vi "Name Msg IO.vi"(4 "IO":T4, 6 "Name Msg":string, 8 "error in":errorcluster, 9 "Name Library File Path":path, 10 "Active Project":refnum<vi>) -> (0 "error out":errorcluster, 2 "Name Msg IO":T1)   [LabVIEW 2025, in "_Rescript.lvlib" / "Msg.lvlib" / "Msg.lvclass"]
uses:
  Msg.lvclass
  IO.ctl
  Name Msg IO.ctl
  Terminal Attributes.ctl
  Attributes.ctl
  <vilib>/Utility/traverseref.llb/TRef TravTarget.ctl
  _Rescript.lvlib
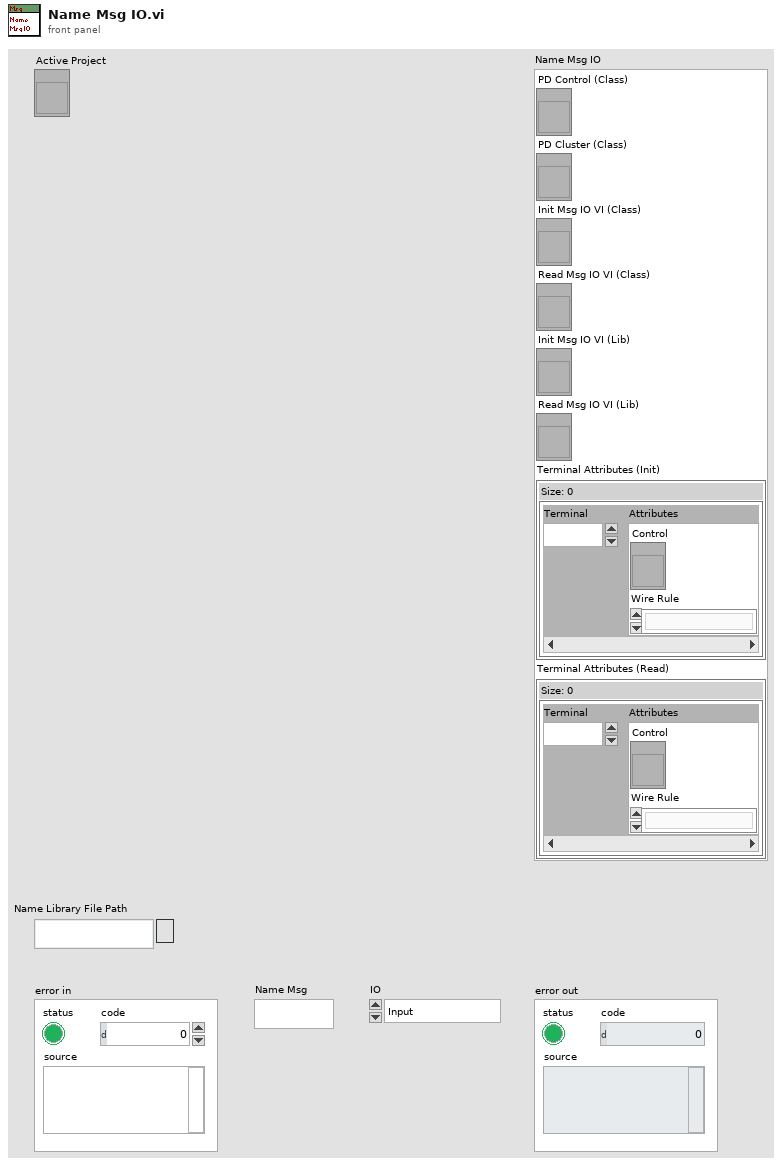
[diagram p1: front panel]
types:
  T1 = typedef "_Rescript.lvlib/Msg.lvlib/Msg.lvclass/Name Msg IO.ctl" = cluster{"PD Control (Class)":refnum<vi>, "PD Cluster (Class)":refnum<vi>, "Init Msg IO VI (Class)":refnum<vi>, "Read Msg IO VI (Class)":refnum<vi>, "Init Msg IO VI (Lib)":refnum<vi>, "Read Msg IO VI (Lib)":refnum<vi>, "Terminal Attributes (Init)":T2, "Terminal Attributes (Read)":T2}
  T2 = typedef "_Rescript.lvlib/Terminal Attributes.ctl" = map{i32, T3}
  T3 = typedef "_Rescript.lvlib/Attributes.ctl" = cluster{"Control":refnum<vi>, "Wire Rule":enum16{"Invalid Wire Rule", "Required", "Recommended", "Optional", "Dynamic Dispatch"}}
  T4 = typedef "_Rescript.lvlib/Msg.lvlib/Msg.lvclass/IO.ctl" = enum16{"Input", "Output"}
  T5 = typedef "TRef TravTarget.ctl" = enum16{"FP", "BD", "Other"}
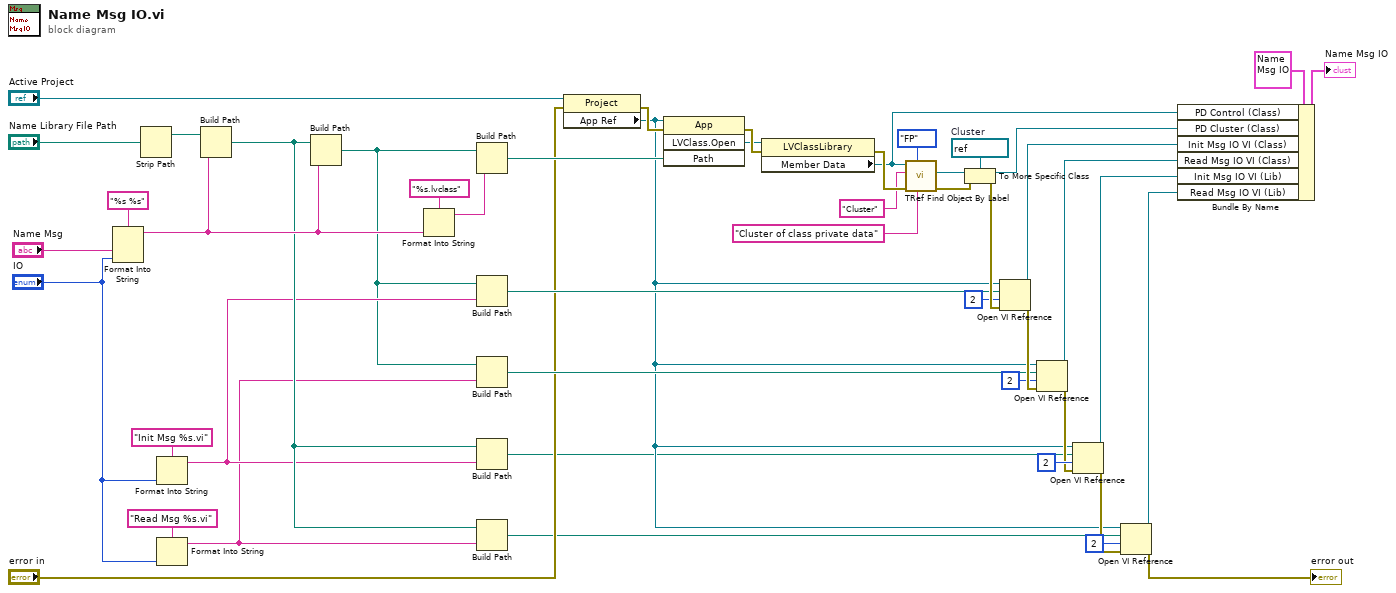
[diagram p0: block diagram]
diagram:
  w43 = refnum<vi> refnum  # Cluster
  n1 = Format Into String(format string="%s %s", "Name Msg", "IO") -> (resulting string=w7:string)  [unwired: 2 in, 1 out]
  n2 = Strip Path(path="Name Library File Path") -> (stripped path=w9:path)  [unwired: 1 out]
  n3 = Format Into String(format string="Init Msg %s.vi", "IO") -> (resulting string=w5:string)  [unwired: 2 in, 1 out]
  n4 = Format Into String(format string="Read Msg %s.vi", "IO") -> (resulting string=w4:string)  [unwired: 2 in, 1 out]
  n5 = Build Path(base path=w9, name or relative path=w7) -> (appended path=w6:path)
  n6 = Build Path(base path=w6, name or relative path=w7) -> (appended path=w1:path)
  n7 = Format Into String(format string="%s.lvclass", w7) -> (resulting string=w36:string)  [unwired: 2 in, 1 out]
  n8 = Build Path(base path=w1, name or relative path=w36) -> (appended path=w37:path)
  n9 = Build Path(base path=w1, name or relative path=w5) -> (appended path=w34:path)
  n10 = Build Path(base path=w1, name or relative path=w4) -> (appended path=w33:path)
  n11 = Build Path(base path=w6, name or relative path=w5) -> (appended path=w3:path)
  n12 = Build Path(base path=w6, name or relative path=w4) -> (appended path=w2:path)
  n13 = property class="Project"(reference="Active Project", error in="error in") -> (error out=w47:errorcluster, "App Ref"=w12:refnum<vi>)  [unwired: 1 out]
  n14 = invoke class="App" method="LVClass.Open"(reference=w12, error in=w47, "Path"=w37) -> (error out=w45:errorcluster, "LVClass.Open"=w38:refnum<vi>)  [unwired: 1 in, 2 out]
  n15 = property class="LVClassLibrary"(reference=w38, error in=w45) -> (error out=w49:errorcluster, "Member Data"=w28:refnum<vi>)  [unwired: 1 out]
  n16 = call <vilib>:"TRef Find Object By Label.vi"("Label"="Cluster of class private data" ("Class Name"), "Traverse Target"=TRef_TravTarget."FP", "error in (no error)"=w49, "Class Name"="Cluster", "VI Ref"=w28) -> ("error out"=w44:errorcluster, "Found Obj Ref"=w42:refnum<vi>)  [unwired: 3 in, 2 out]
  n17 = To More Specific Class(target class=w43, reference=w42, error in=w44) -> (specific class reference=w27:refnum<vi>, error out=w46:errorcluster)
  n18 = Open VI Reference(application reference (local)=w12, vi path=w34, options=2, error in (no error)=w46) -> (vi reference=w26:refnum<vi>, error out=w48:errorcluster)  [unwired: 2 in]
  n19 = Open VI Reference(application reference (local)=w12, vi path=w33, options=2, error in (no error)=w48) -> (vi reference=w25:refnum<vi>, error out=w14:errorcluster)  [unwired: 2 in]
  n20 = Open VI Reference(application reference (local)=w12, vi path=w3, options=2, error in (no error)=w14) -> (vi reference=w11:refnum<vi>, error out=w15:errorcluster)  [unwired: 2 in]
  n21 = Open VI Reference(application reference (local)=w12, vi path=w2, options=2, error in (no error)=w15) -> (vi reference=w10:refnum<vi>, error out=→"error out":errorcluster)  [unwired: 2 in]
  n22 = Bundle By Name(cluster=T1 {"PD Control (Class)"=refnum, "PD Cluster (Class)"=refnum, "Init Msg IO VI (Class)"=refnum, "Read Msg IO VI (Class)"=refnum, "Init Msg IO VI (Lib)"=refnum, "Read Msg IO VI (Lib)"=refnum, "Terminal Attributes (Init)"={}, "Terminal Attributes (Read)"={}} ("Name Msg IO"), "PD Control (Class)"=w28, "PD Cluster (Class)"=w27, "Init Msg IO VI (Class)"=w26, "Read Msg IO VI (Class)"=w25, "Init Msg IO VI (Lib)"=w11, "Read Msg IO VI (Lib)"=w10) -> (→"Name Msg IO":T1)
